vi "Format IDCol.vi"(10 "ID Format":u16(ring) caption="ID格式" items=["十六进制", "十进制"], 11 "Data":T1 {"Direction" items=["Tx", "Rx"]; "CANType" items=["CAN", "CANFD", "CANFD加速"]}) -> (3 "ID str":string)   [LabVIEW 2011, in "CAN FD.lvlib"]
uses:
  CAN FD.lvlib
  Typedef/CAN Data.ctl
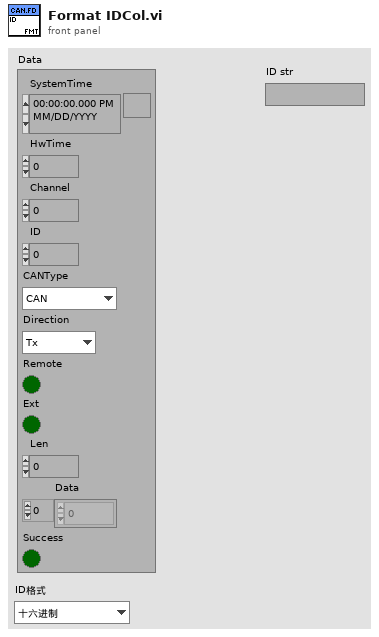
[diagram p1: front panel]
types:
  T1 = typedef "CAN FD.lvlib/CAN Data.ctl" = cluster{"SystemTime":timestamp, "HwTime":dbl, "Channel":u8, "ID":u32, "CANType":i16, "Direction":i16, "Remote":bool, "Ext":bool, "Len":u8, "Data":u8[], "Success":bool}
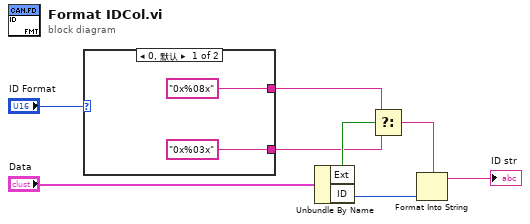
[diagram p0: block diagram]
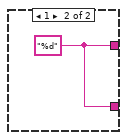
[diagram p2: hidden frame]
diagram:
  n1 = case shown="0, 默认" "ID Format" {
    tunnel: ["0x%08x" ("格式字符串") w11] -> w5
    tunnel: ["0x%03x" ("格式字符串") w11] -> w4
    frame 0, Default {
    }
    frame 1 {
      w11 = "%d" ("格式字符串")
    }
  }
  n2 = Unbundle By Name("Data") -> ("Ext"=w7:bool, "ID"=w8:u32)
  n3 = Select(t=w5, s=w7, f=w4) -> (s? t:f=w6:string)
  n4 = Format Into String(format string=w6, w8) -> (resulting string=→"ID str":string)  [unwired: 2 in, 1 out]
